vi "List Root Test ID.vi"(8 "error in (no error)":errorcluster, 11 "Test Executive in":refnum<class "Test Executive.lvclass">) -> (0 "error out":errorcluster, 3 "Test Executive out":refnum<class "Test Executive.lvclass">, 4 "Root IDs":string[](array[string]), 5 "Root ID":string, 6 "Root Names":string[](array[string]))   [LabVIEW 2017, in "Test Executive.lvlib" / "Test Executive.lvclass"]
uses:
  <vilib>/gpm_packages/@cs/test-executive/Source/Test Executive/TestExecutive/Test Executive.lvclass
  <vilib>/gpm_packages/@cs/test-executive/Source/Test Executive/TestExecutive/Test Executive.lvclass/Test Executive.ctl
  <vilib>/gpm_packages/@cs/linked-list/Source/Linked List/Linked List Ref/Linked List Ref.lvclass
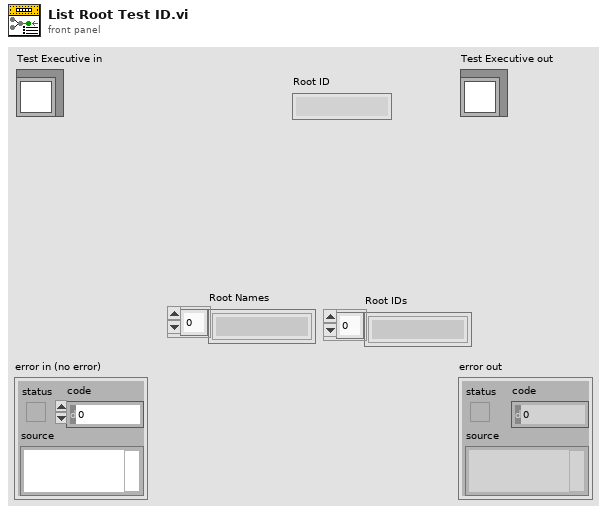
[diagram p1: front panel]
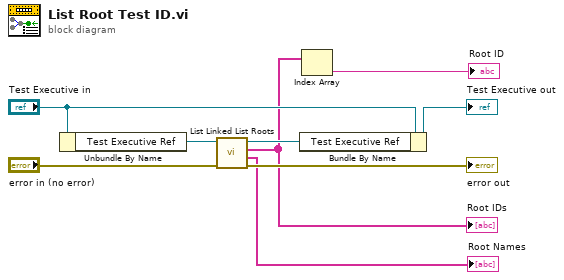
[diagram p0: block diagram]
diagram:
  n1 = Unbundle By Name("Test Executive in") -> ("Test Executive Ref"=w9:refnum<data-value>)
  n2 = call <vilib>:"List Linked List Roots.vi"("error in (no error)"="error in (no error)", "Linked List Ref"=w9) -> ("error out"=→"error out":errorcluster, "Root Names"=→"Root Names":string[], "Root IDs"=w3:string[], "Linked List Ref out"=w7:refnum<data-value>)  [unwired: 6 in]
  "Root IDs" <- w3
  n3 = Bundle By Name(cluster="Test Executive in", "Test Executive Ref"=w7) -> (→"Test Executive out":refnum<class "Test Executive.lvclass">)
  n4 = Index Array(array=w3) -> (element=→"Root ID":string)  [unwired: 1 in]
